vi "Sub-VI 1.vi"(0 "Select the chord name":string(combo), 1 "Display the musical notes":bool caption="Display the musical notes ?", 2 "Stop conversion":bool) -> (4 "B11":bool caption="Boolean", 8 "B1":bool caption="Boolean", 9 "N1":bool, 10 "B2":bool caption="Boolean", 11 "N2":bool, 12 "B3":bool caption="Boolean", 13 "N3":bool, 14 "B4":bool caption="Boolean", 15 "N4":bool, 16 "B5":bool caption="Boolean", 17 "N5":bool, 18 "B6":bool caption="Boolean", 19 "N6":bool, 20 "B7":bool caption="Boolean", 21 "B8":bool caption="Boolean", 22 "B9":bool caption="Boolean", 23 "B10":bool caption="Boolean", 26 "N7":bool, 27 "N8":bool)   [LabVIEW 2019]
panel:
  # "CHORDS BOX"
  # "Welcome \ndear apprentices"
  # "This App, tailor-made for you, has magic power. Which ?  \n\nThat of making you travel in the shoes \nof one of the greatest pianists of all time :"
  # "NOTES PLAYED BOX"
  # "3"
  # "4"
  # "5"
  # "6"
  # "7"
  # "1"
  # "2"
  # "8"
  # "Sir Elton John."
  # "Let yourself \nbe transported by its chords !"
  # "2"
  # "3"
  # "4"
  # "5"
  # "6"
  # "8"
  # "1"
  # "7"
  # "9"
  # "10"
  # "11"
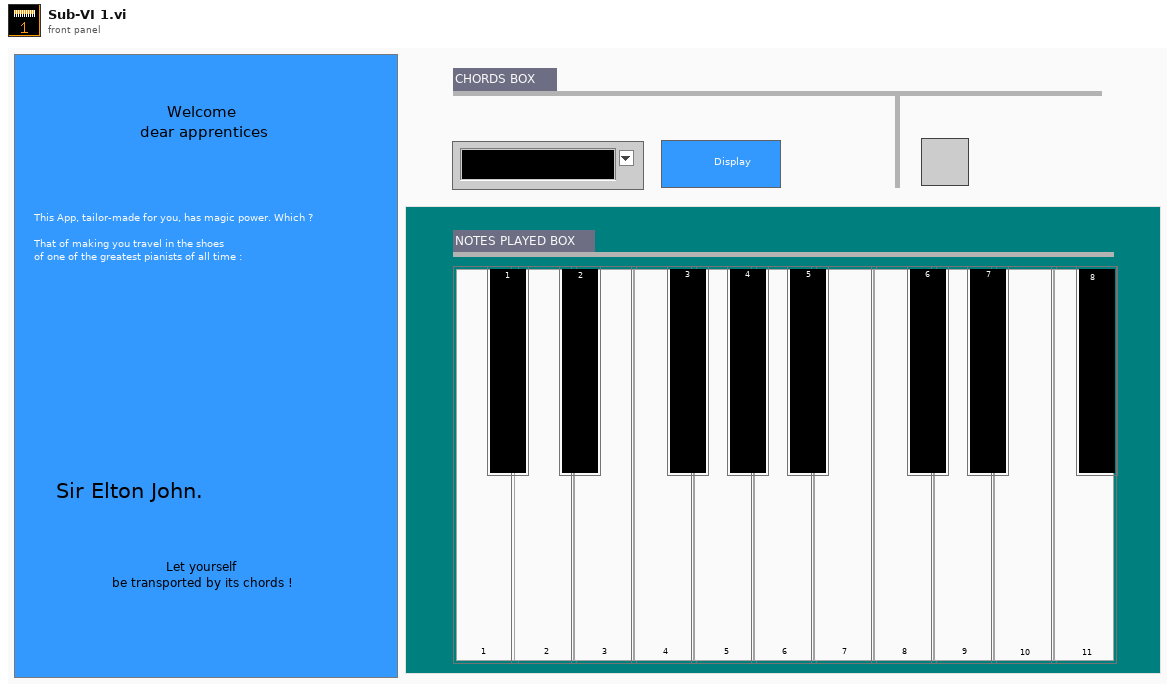
[diagram p1: front panel]
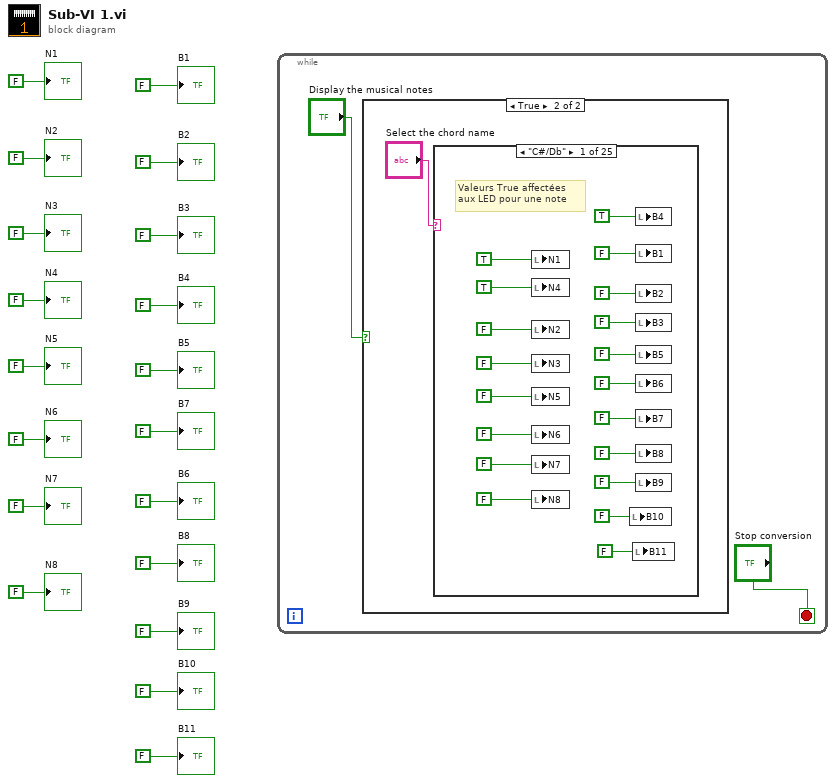
[diagram p0: block diagram]
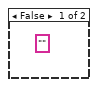
[diagram p2: hidden frame]
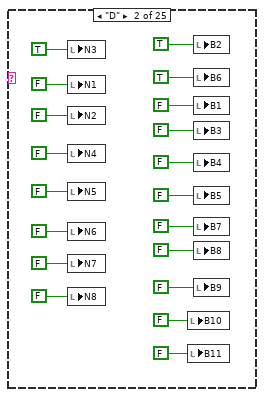
[diagram p3: hidden frame]
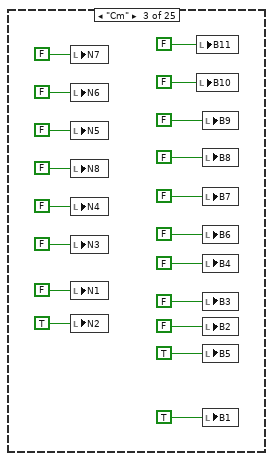
[diagram p4: hidden frame]
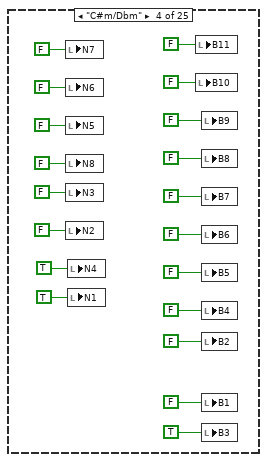
[diagram p5: hidden frame]
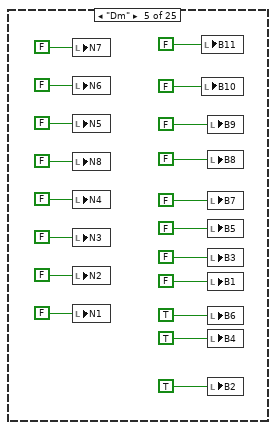
[diagram p6: hidden frame]
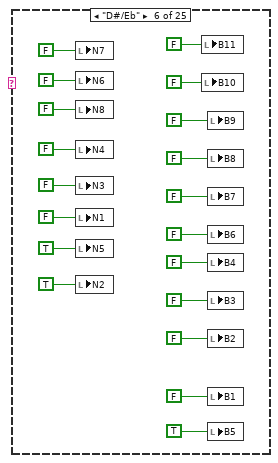
[diagram p7: hidden frame]
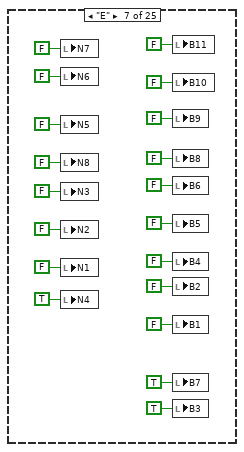
[diagram p8: hidden frame]
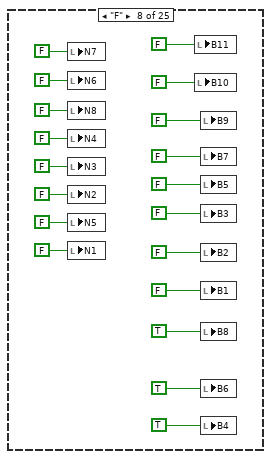
[diagram p9: hidden frame]
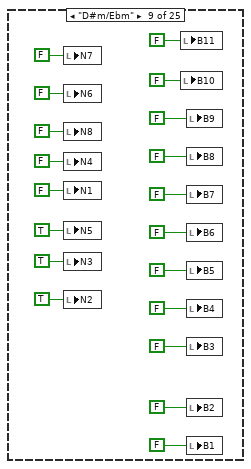
[diagram p10: hidden frame]
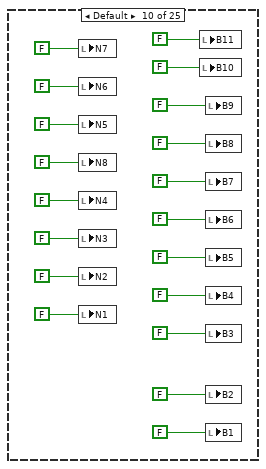
[diagram p11: hidden frame]
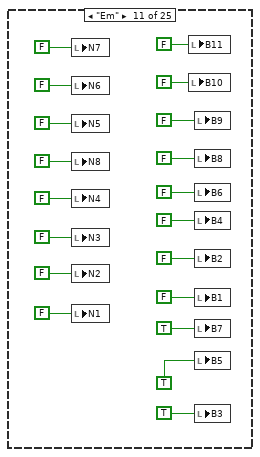
[diagram p12: hidden frame]
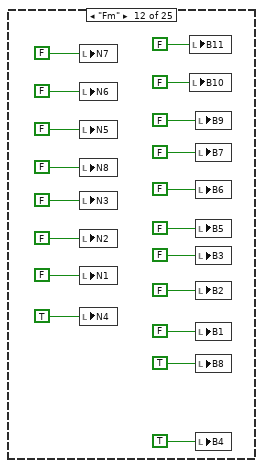
[diagram p13: hidden frame]
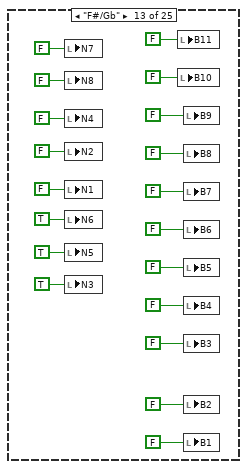
[diagram p14: hidden frame]
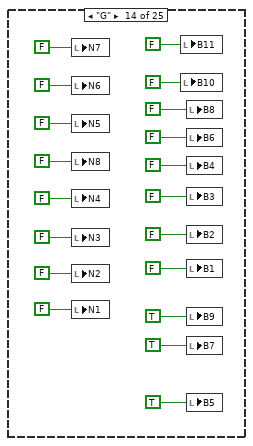
[diagram p15: hidden frame]
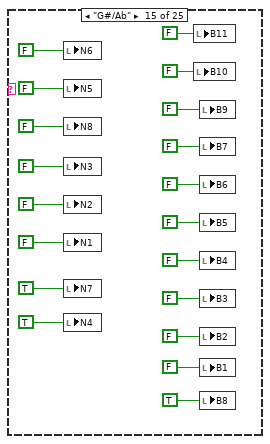
[diagram p16: hidden frame]
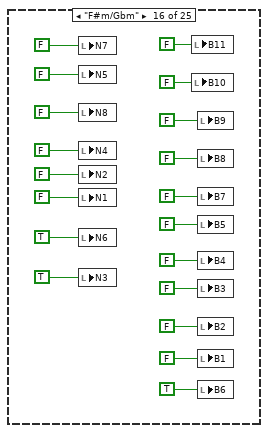
[diagram p17: hidden frame]
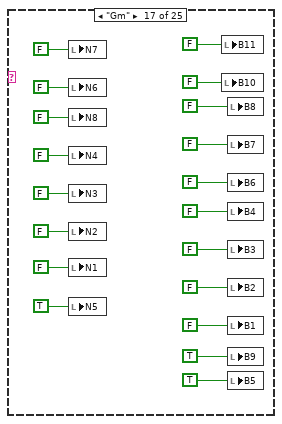
[diagram p18: hidden frame]
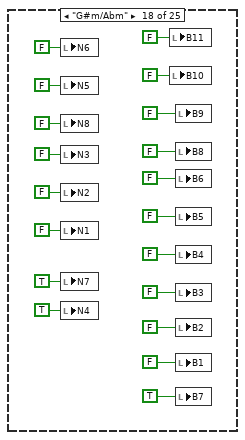
[diagram p19: hidden frame]
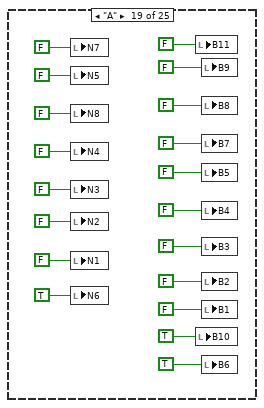
[diagram p20: hidden frame]
diagram:
  n1 = while {
    stop <- "Stop conversion" stop-if-true
    n2 = case shown="True" "Display the musical notes" {
      frame False {
        (unwired) ""
      }
      frame True {
        n3 = case shown="\"C#/Db\"" "Select the chord name" {
          frame "C#/Db" {
            # "Valeurs True affectées\naux LED pour une note"
            n4 = local write "N1"(TRUE) -> ()
            n5 = local write "N4"(TRUE) -> ()
            n6 = local write "N2"(FALSE) -> ()
            n7 = local write "N3"(FALSE) -> ()
            n8 = local write "N5"(FALSE) -> ()
            n9 = local write "N6"(FALSE) -> ()
            n10 = local write "N7"(FALSE) -> ()
            n11 = local write "N8"(FALSE) -> ()
            n12 = local write "B10"(FALSE) -> ()
            n13 = local write "B11"(FALSE) -> ()
            n14 = local write "B4"(TRUE) -> ()
            n15 = local write "B1"(FALSE) -> ()
            n16 = local write "B2"(FALSE) -> ()
            n17 = local write "B3"(FALSE) -> ()
            n18 = local write "B5"(FALSE) -> ()
            n19 = local write "B6"(FALSE) -> ()
            n20 = local write "B7"(FALSE) -> ()
            n21 = local write "B8"(FALSE) -> ()
            n22 = local write "B9"(FALSE) -> ()
          }
          frame "D" {
            n23 = local write "N3"(TRUE) -> ()
            n24 = local write "N1"(FALSE) -> ()
            n25 = local write "N2"(FALSE) -> ()
            n26 = local write "N4"(FALSE) -> ()
            n27 = local write "N5"(FALSE) -> ()
            n28 = local write "N6"(FALSE) -> ()
            n29 = local write "N7"(FALSE) -> ()
            n30 = local write "N8"(FALSE) -> ()
            n31 = local write "B10"(FALSE) -> ()
            n32 = local write "B11"(FALSE) -> ()
            n33 = local write "B2"(TRUE) -> ()
            n34 = local write "B6"(TRUE) -> ()
            n35 = local write "B1"(FALSE) -> ()
            n36 = local write "B3"(FALSE) -> ()
            n37 = local write "B4"(FALSE) -> ()
            n38 = local write "B5"(FALSE) -> ()
            n39 = local write "B7"(FALSE) -> ()
            n40 = local write "B8"(FALSE) -> ()
            n41 = local write "B9"(FALSE) -> ()
          }
          frame "Cm" {
            n42 = local write "N7"(FALSE) -> ()
            n43 = local write "N6"(FALSE) -> ()
            n44 = local write "N5"(FALSE) -> ()
            n45 = local write "N8"(FALSE) -> ()
            n46 = local write "N4"(FALSE) -> ()
            n47 = local write "N3"(FALSE) -> ()
            n48 = local write "N1"(FALSE) -> ()
            n49 = local write "N2"(TRUE) -> ()
            n50 = local write "B11"(FALSE) -> ()
            n51 = local write "B10"(FALSE) -> ()
            n52 = local write "B9"(FALSE) -> ()
            n53 = local write "B8"(FALSE) -> ()
            n54 = local write "B7"(FALSE) -> ()
            n55 = local write "B6"(FALSE) -> ()
            n56 = local write "B4"(FALSE) -> ()
            n57 = local write "B3"(FALSE) -> ()
            n58 = local write "B2"(FALSE) -> ()
            n59 = local write "B5"(TRUE) -> ()
            n60 = local write "B1"(TRUE) -> ()
          }
          frame "C#m/Dbm" {
            n61 = local write "N7"(FALSE) -> ()
            n62 = local write "N6"(FALSE) -> ()
            n63 = local write "N5"(FALSE) -> ()
            n64 = local write "N8"(FALSE) -> ()
            n65 = local write "N3"(FALSE) -> ()
            n66 = local write "N2"(FALSE) -> ()
            n67 = local write "N4"(TRUE) -> ()
            n68 = local write "N1"(TRUE) -> ()
            n69 = local write "B11"(FALSE) -> ()
            n70 = local write "B10"(FALSE) -> ()
            n71 = local write "B9"(FALSE) -> ()
            n72 = local write "B8"(FALSE) -> ()
            n73 = local write "B7"(FALSE) -> ()
            n74 = local write "B6"(FALSE) -> ()
            n75 = local write "B5"(FALSE) -> ()
            n76 = local write "B4"(FALSE) -> ()
            n77 = local write "B2"(FALSE) -> ()
            n78 = local write "B1"(FALSE) -> ()
            n79 = local write "B3"(TRUE) -> ()
          }
          frame "Dm" {
            n80 = local write "N7"(FALSE) -> ()
            n81 = local write "N6"(FALSE) -> ()
            n82 = local write "N5"(FALSE) -> ()
            n83 = local write "N8"(FALSE) -> ()
            n84 = local write "N4"(FALSE) -> ()
            n85 = local write "N3"(FALSE) -> ()
            n86 = local write "N2"(FALSE) -> ()
            n87 = local write "N1"(FALSE) -> ()
            n88 = local write "B11"(FALSE) -> ()
            n89 = local write "B10"(FALSE) -> ()
            n90 = local write "B9"(FALSE) -> ()
            n91 = local write "B8"(FALSE) -> ()
            n92 = local write "B7"(FALSE) -> ()
            n93 = local write "B5"(FALSE) -> ()
            n94 = local write "B3"(FALSE) -> ()
            n95 = local write "B1"(FALSE) -> ()
            n96 = local write "B6"(TRUE) -> ()
            n97 = local write "B4"(TRUE) -> ()
            n98 = local write "B2"(TRUE) -> ()
          }
          frame "D#/Eb" {
            n99 = local write "N7"(FALSE) -> ()
            n100 = local write "N6"(FALSE) -> ()
            n101 = local write "N8"(FALSE) -> ()
            n102 = local write "N4"(FALSE) -> ()
            n103 = local write "N3"(FALSE) -> ()
            n104 = local write "N1"(FALSE) -> ()
            n105 = local write "N5"(TRUE) -> ()
            n106 = local write "N2"(TRUE) -> ()
            n107 = local write "B11"(FALSE) -> ()
            n108 = local write "B10"(FALSE) -> ()
            n109 = local write "B9"(FALSE) -> ()
            n110 = local write "B8"(FALSE) -> ()
            n111 = local write "B7"(FALSE) -> ()
            n112 = local write "B6"(FALSE) -> ()
            n113 = local write "B4"(FALSE) -> ()
            n114 = local write "B3"(FALSE) -> ()
            n115 = local write "B2"(FALSE) -> ()
            n116 = local write "B1"(FALSE) -> ()
            n117 = local write "B5"(TRUE) -> ()
          }
          frame "E" {
            n118 = local write "N7"(FALSE) -> ()
            n119 = local write "N6"(FALSE) -> ()
            n120 = local write "N5"(FALSE) -> ()
            n121 = local write "N8"(FALSE) -> ()
            n122 = local write "N3"(FALSE) -> ()
            n123 = local write "N2"(FALSE) -> ()
            n124 = local write "N1"(FALSE) -> ()
            n125 = local write "N4"(TRUE) -> ()
            n126 = local write "B11"(FALSE) -> ()
            n127 = local write "B10"(FALSE) -> ()
            n128 = local write "B9"(FALSE) -> ()
            n129 = local write "B8"(FALSE) -> ()
            n130 = local write "B6"(FALSE) -> ()
            n131 = local write "B5"(FALSE) -> ()
            n132 = local write "B4"(FALSE) -> ()
            n133 = local write "B2"(FALSE) -> ()
            n134 = local write "B1"(FALSE) -> ()
            n135 = local write "B7"(TRUE) -> ()
            n136 = local write "B3"(TRUE) -> ()
          }
          frame "F" {
            n137 = local write "N7"(FALSE) -> ()
            n138 = local write "N6"(FALSE) -> ()
            n139 = local write "N8"(FALSE) -> ()
            n140 = local write "N4"(FALSE) -> ()
            n141 = local write "N3"(FALSE) -> ()
            n142 = local write "N2"(FALSE) -> ()
            n143 = local write "N5"(FALSE) -> ()
            n144 = local write "N1"(FALSE) -> ()
            n145 = local write "B11"(FALSE) -> ()
            n146 = local write "B10"(FALSE) -> ()
            n147 = local write "B9"(FALSE) -> ()
            n148 = local write "B7"(FALSE) -> ()
            n149 = local write "B5"(FALSE) -> ()
            n150 = local write "B3"(FALSE) -> ()
            n151 = local write "B2"(FALSE) -> ()
            n152 = local write "B1"(FALSE) -> ()
            n153 = local write "B8"(TRUE) -> ()
            n154 = local write "B6"(TRUE) -> ()
            n155 = local write "B4"(TRUE) -> ()
          }
          frame "D#m/Ebm" {
            n156 = local write "N7"(FALSE) -> ()
            n157 = local write "N6"(FALSE) -> ()
            n158 = local write "N8"(FALSE) -> ()
            n159 = local write "N4"(FALSE) -> ()
            n160 = local write "N1"(FALSE) -> ()
            n161 = local write "N5"(TRUE) -> ()
            n162 = local write "N3"(TRUE) -> ()
            n163 = local write "N2"(TRUE) -> ()
            n164 = local write "B11"(FALSE) -> ()
            n165 = local write "B10"(FALSE) -> ()
            n166 = local write "B9"(FALSE) -> ()
            n167 = local write "B8"(FALSE) -> ()
            n168 = local write "B7"(FALSE) -> ()
            n169 = local write "B6"(FALSE) -> ()
            n170 = local write "B5"(FALSE) -> ()
            n171 = local write "B4"(FALSE) -> ()
            n172 = local write "B3"(FALSE) -> ()
            n173 = local write "B2"(FALSE) -> ()
            n174 = local write "B1"(FALSE) -> ()
          }
          frame Default {
            n175 = local write "N7"(FALSE) -> ()
            n176 = local write "N6"(FALSE) -> ()
            n177 = local write "N5"(FALSE) -> ()
            n178 = local write "N8"(FALSE) -> ()
            n179 = local write "N4"(FALSE) -> ()
            n180 = local write "N3"(FALSE) -> ()
            n181 = local write "N2"(FALSE) -> ()
            n182 = local write "N1"(FALSE) -> ()
            n183 = local write "B11"(FALSE) -> ()
            n184 = local write "B10"(FALSE) -> ()
            n185 = local write "B9"(FALSE) -> ()
            n186 = local write "B8"(FALSE) -> ()
            n187 = local write "B7"(FALSE) -> ()
            n188 = local write "B6"(FALSE) -> ()
            n189 = local write "B5"(FALSE) -> ()
            n190 = local write "B4"(FALSE) -> ()
            n191 = local write "B3"(FALSE) -> ()
            n192 = local write "B2"(FALSE) -> ()
            n193 = local write "B1"(FALSE) -> ()
          }
          frame "Em" {
            n194 = local write "N7"(FALSE) -> ()
            n195 = local write "N6"(FALSE) -> ()
            n196 = local write "N5"(FALSE) -> ()
            n197 = local write "N8"(FALSE) -> ()
            n198 = local write "N4"(FALSE) -> ()
            n199 = local write "N3"(FALSE) -> ()
            n200 = local write "N2"(FALSE) -> ()
            n201 = local write "N1"(FALSE) -> ()
            n202 = local write "B11"(FALSE) -> ()
            n203 = local write "B10"(FALSE) -> ()
            n204 = local write "B9"(FALSE) -> ()
            n205 = local write "B8"(FALSE) -> ()
            n206 = local write "B6"(FALSE) -> ()
            n207 = local write "B4"(FALSE) -> ()
            n208 = local write "B2"(FALSE) -> ()
            n209 = local write "B1"(FALSE) -> ()
            n210 = local write "B7"(TRUE) -> ()
            n211 = local write "B5"(TRUE) -> ()
            n212 = local write "B3"(TRUE) -> ()
          }
          frame "Fm" {
            n213 = local write "N7"(FALSE) -> ()
            n214 = local write "N6"(FALSE) -> ()
            n215 = local write "N5"(FALSE) -> ()
            n216 = local write "N8"(FALSE) -> ()
            n217 = local write "N3"(FALSE) -> ()
            n218 = local write "N2"(FALSE) -> ()
            n219 = local write "N1"(FALSE) -> ()
            n220 = local write "N4"(TRUE) -> ()
            n221 = local write "B11"(FALSE) -> ()
            n222 = local write "B10"(FALSE) -> ()
            n223 = local write "B9"(FALSE) -> ()
            n224 = local write "B7"(FALSE) -> ()
            n225 = local write "B6"(FALSE) -> ()
            n226 = local write "B5"(FALSE) -> ()
            n227 = local write "B3"(FALSE) -> ()
            n228 = local write "B2"(FALSE) -> ()
            n229 = local write "B1"(FALSE) -> ()
            n230 = local write "B8"(TRUE) -> ()
            n231 = local write "B4"(TRUE) -> ()
          }
          frame "F#/Gb" {
            n232 = local write "N7"(FALSE) -> ()
            n233 = local write "N8"(FALSE) -> ()
            n234 = local write "N4"(FALSE) -> ()
            n235 = local write "N2"(FALSE) -> ()
            n236 = local write "N1"(FALSE) -> ()
            n237 = local write "N6"(TRUE) -> ()
            n238 = local write "N5"(TRUE) -> ()
            n239 = local write "N3"(TRUE) -> ()
            n240 = local write "B11"(FALSE) -> ()
            n241 = local write "B10"(FALSE) -> ()
            n242 = local write "B9"(FALSE) -> ()
            n243 = local write "B8"(FALSE) -> ()
            n244 = local write "B7"(FALSE) -> ()
            n245 = local write "B6"(FALSE) -> ()
            n246 = local write "B5"(FALSE) -> ()
            n247 = local write "B4"(FALSE) -> ()
            n248 = local write "B3"(FALSE) -> ()
            n249 = local write "B2"(FALSE) -> ()
            n250 = local write "B1"(FALSE) -> ()
          }
          frame "G" {
            n251 = local write "N7"(FALSE) -> ()
            n252 = local write "N6"(FALSE) -> ()
            n253 = local write "N5"(FALSE) -> ()
            n254 = local write "N8"(FALSE) -> ()
            n255 = local write "N4"(FALSE) -> ()
            n256 = local write "N3"(FALSE) -> ()
            n257 = local write "N2"(FALSE) -> ()
            n258 = local write "N1"(FALSE) -> ()
            n259 = local write "B11"(FALSE) -> ()
            n260 = local write "B10"(FALSE) -> ()
            n261 = local write "B8"(FALSE) -> ()
            n262 = local write "B6"(FALSE) -> ()
            n263 = local write "B4"(FALSE) -> ()
            n264 = local write "B3"(FALSE) -> ()
            n265 = local write "B2"(FALSE) -> ()
            n266 = local write "B1"(FALSE) -> ()
            n267 = local write "B9"(TRUE) -> ()
            n268 = local write "B7"(TRUE) -> ()
            n269 = local write "B5"(TRUE) -> ()
          }
          frame "G#/Ab" {
            n270 = local write "N6"(FALSE) -> ()
            n271 = local write "N5"(FALSE) -> ()
            n272 = local write "N8"(FALSE) -> ()
            n273 = local write "N3"(FALSE) -> ()
            n274 = local write "N2"(FALSE) -> ()
            n275 = local write "N1"(FALSE) -> ()
            n276 = local write "N7"(TRUE) -> ()
            n277 = local write "N4"(TRUE) -> ()
            n278 = local write "B11"(FALSE) -> ()
            n279 = local write "B10"(FALSE) -> ()
            n280 = local write "B9"(FALSE) -> ()
            n281 = local write "B7"(FALSE) -> ()
            n282 = local write "B6"(FALSE) -> ()
            n283 = local write "B5"(FALSE) -> ()
            n284 = local write "B4"(FALSE) -> ()
            n285 = local write "B3"(FALSE) -> ()
            n286 = local write "B2"(FALSE) -> ()
            n287 = local write "B1"(FALSE) -> ()
            n288 = local write "B8"(TRUE) -> ()
          }
          frame "F#m/Gbm" {
            n289 = local write "N7"(FALSE) -> ()
            n290 = local write "N5"(FALSE) -> ()
            n291 = local write "N8"(FALSE) -> ()
            n292 = local write "N4"(FALSE) -> ()
            n293 = local write "N2"(FALSE) -> ()
            n294 = local write "N1"(FALSE) -> ()
            n295 = local write "N6"(TRUE) -> ()
            n296 = local write "N3"(TRUE) -> ()
            n297 = local write "B11"(FALSE) -> ()
            n298 = local write "B10"(FALSE) -> ()
            n299 = local write "B9"(FALSE) -> ()
            n300 = local write "B8"(FALSE) -> ()
            n301 = local write "B7"(FALSE) -> ()
            n302 = local write "B5"(FALSE) -> ()
            n303 = local write "B4"(FALSE) -> ()
            n304 = local write "B3"(FALSE) -> ()
            n305 = local write "B2"(FALSE) -> ()
            n306 = local write "B1"(FALSE) -> ()
            n307 = local write "B6"(TRUE) -> ()
          }
          frame "Gm" {
            n308 = local write "N7"(FALSE) -> ()
            n309 = local write "N6"(FALSE) -> ()
            n310 = local write "N8"(FALSE) -> ()
            n311 = local write "N4"(FALSE) -> ()
            n312 = local write "N3"(FALSE) -> ()
            n313 = local write "N2"(FALSE) -> ()
            n314 = local write "N1"(FALSE) -> ()
            n315 = local write "N5"(TRUE) -> ()
            n316 = local write "B11"(FALSE) -> ()
            n317 = local write "B10"(FALSE) -> ()
            n318 = local write "B8"(FALSE) -> ()
            n319 = local write "B7"(FALSE) -> ()
            n320 = local write "B6"(FALSE) -> ()
            n321 = local write "B4"(FALSE) -> ()
            n322 = local write "B3"(FALSE) -> ()
            n323 = local write "B2"(FALSE) -> ()
            n324 = local write "B1"(FALSE) -> ()
            n325 = local write "B9"(TRUE) -> ()
            n326 = local write "B5"(TRUE) -> ()
          }
          frame "G#m/Abm" {
            n327 = local write "N6"(FALSE) -> ()
            n328 = local write "N5"(FALSE) -> ()
            n329 = local write "N8"(FALSE) -> ()
            n330 = local write "N3"(FALSE) -> ()
            n331 = local write "N2"(FALSE) -> ()
            n332 = local write "N1"(FALSE) -> ()
            n333 = local write "N7"(TRUE) -> ()
            n334 = local write "N4"(TRUE) -> ()
            n335 = local write "B11"(FALSE) -> ()
            n336 = local write "B10"(FALSE) -> ()
            n337 = local write "B9"(FALSE) -> ()
            n338 = local write "B8"(FALSE) -> ()
            n339 = local write "B6"(FALSE) -> ()
            n340 = local write "B5"(FALSE) -> ()
            n341 = local write "B4"(FALSE) -> ()
            n342 = local write "B3"(FALSE) -> ()
            n343 = local write "B2"(FALSE) -> ()
            n344 = local write "B1"(FALSE) -> ()
            n345 = local write "B7"(TRUE) -> ()
          }
          frame "A" {
            n346 = local write "N7"(FALSE) -> ()
            n347 = local write "N5"(FALSE) -> ()
            n348 = local write "N8"(FALSE) -> ()
            n349 = local write "N4"(FALSE) -> ()
            n350 = local write "N3"(FALSE) -> ()
            n351 = local write "N2"(FALSE) -> ()
            n352 = local write "N1"(FALSE) -> ()
            n353 = local write "N6"(TRUE) -> ()
            n354 = local write "B11"(FALSE) -> ()
            n355 = local write "B10"(TRUE) -> ()
            n356 = local write "B9"(FALSE) -> ()
            n357 = local write "B8"(FALSE) -> ()
            n358 = local write "B7"(FALSE) -> ()
            n359 = local write "B5"(FALSE) -> ()
            n360 = local write "B4"(FALSE) -> ()
            n361 = local write "B3"(FALSE) -> ()
            n362 = local write "B2"(FALSE) -> ()
            n363 = local write "B1"(FALSE) -> ()
            n364 = local write "B6"(TRUE) -> ()
          }
          frame "A#/Bb" {
            n365 = local write "N8"(FALSE) -> ()
            n366 = local write "N4"(FALSE) -> ()
            n367 = local write "N3"(FALSE) -> ()
            n368 = local write "N2"(FALSE) -> ()
            n369 = local write "N1"(FALSE) -> ()
            n370 = local write "N5"(TRUE) -> ()
            n371 = local write "B10"(FALSE) -> ()
            n372 = local write "B11"(TRUE) -> ()
            n373 = local write "B8"(FALSE) -> ()
            n374 = local write "B7"(FALSE) -> ()
            n375 = local write "B6"(FALSE) -> ()
            n376 = local write "B5"(FALSE) -> ()
            n377 = local write "B4"(FALSE) -> ()
            n378 = local write "B3"(FALSE) -> ()
            n379 = local write "B2"(FALSE) -> ()
            n380 = local write "B1"(FALSE) -> ()
            n381 = local write "B9"(TRUE) -> ()
          }
          frame "B" {
            n382 = local write "N6"(FALSE) -> ()
            n383 = local write "N5"(FALSE) -> ()
            n384 = local write "N4"(FALSE) -> ()
            n385 = local write "N3"(FALSE) -> ()
            n386 = local write "N2"(FALSE) -> ()
            n387 = local write "N1"(FALSE) -> ()
            n388 = local write "N7"(TRUE) -> ()
            n389 = local write "N8"(TRUE) -> ()
            n390 = local write "B11"(FALSE) -> ()
            n391 = local write "B10"(FALSE) -> ()
            n392 = local write "B9"(FALSE) -> ()
            n393 = local write "B8"(FALSE) -> ()
            n394 = local write "B6"(FALSE) -> ()
            n395 = local write "B5"(FALSE) -> ()
            n396 = local write "B4"(FALSE) -> ()
            n397 = local write "B3"(FALSE) -> ()
            n398 = local write "B2"(FALSE) -> ()
            n399 = local write "B1"(FALSE) -> ()
            n400 = local write "B7"(TRUE) -> ()
          }
          frame "Am" {
            n401 = local write "N7"(FALSE) -> ()
            n402 = local write "N6"(FALSE) -> ()
            n403 = local write "N5"(FALSE) -> ()
            n404 = local write "N8"(FALSE) -> ()
            n405 = local write "N4"(FALSE) -> ()
            n406 = local write "N3"(FALSE) -> ()
            n407 = local write "N2"(FALSE) -> ()
            n408 = local write "N1"(FALSE) -> ()
            n409 = local write "B11"(FALSE) -> ()
            n410 = local write "B10"(TRUE) -> ()
            n411 = local write "B9"(FALSE) -> ()
            n412 = local write "B7"(FALSE) -> ()
            n413 = local write "B5"(FALSE) -> ()
            n414 = local write "B4"(FALSE) -> ()
            n415 = local write "B3"(FALSE) -> ()
            n416 = local write "B2"(FALSE) -> ()
            n417 = local write "B1"(FALSE) -> ()
            n418 = local write "B8"(TRUE) -> ()
            n419 = local write "B6"(TRUE) -> ()
          }
          frame "A#m/Bbm" {
            n420 = local write "N7"(FALSE) -> ()
            n421 = local write "N8"(FALSE) -> ()
            n422 = local write "N4"(FALSE) -> ()
            n423 = local write "N3"(FALSE) -> ()
            n424 = local write "N2"(FALSE) -> ()
            n425 = local write "N1"(FALSE) -> ()
            n426 = local write "N6"(TRUE) -> ()
            n427 = local write "N5"(TRUE) -> ()
            n428 = local write "B10"(FALSE) -> ()
            n429 = local write "B11"(TRUE) -> ()
            n430 = local write "B9"(FALSE) -> ()
            n431 = local write "B8"(FALSE) -> ()
            n432 = local write "B7"(FALSE) -> ()
            n433 = local write "B6"(FALSE) -> ()
            n434 = local write "B5"(FALSE) -> ()
            n435 = local write "B4"(FALSE) -> ()
            n436 = local write "B3"(FALSE) -> ()
            n437 = local write "B2"(FALSE) -> ()
            n438 = local write "B1"(FALSE) -> ()
          }
          frame "Bm" {
            n439 = local write "N7"(FALSE) -> ()
            n440 = local write "N6"(FALSE) -> ()
            n441 = local write "N5"(FALSE) -> ()
            n442 = local write "N4"(FALSE) -> ()
            n443 = local write "N3"(FALSE) -> ()
            n444 = local write "N2"(FALSE) -> ()
            n445 = local write "N1"(FALSE) -> ()
            n446 = local write "N8"(TRUE) -> ()
            n447 = local write "B11"(FALSE) -> ()
            n448 = local write "B10"(FALSE) -> ()
            n449 = local write "B8"(FALSE) -> ()
            n450 = local write "B6"(FALSE) -> ()
            n451 = local write "B5"(FALSE) -> ()
            n452 = local write "B4"(FALSE) -> ()
            n453 = local write "B3"(FALSE) -> ()
            n454 = local write "B2"(FALSE) -> ()
            n455 = local write "B1"(FALSE) -> ()
            n456 = local write "B9"(TRUE) -> ()
            n457 = local write "B7"(TRUE) -> ()
          }
          frame "C" {
            n458 = local write "N7"(FALSE) -> ()
            n459 = local write "N6"(FALSE) -> ()
            n460 = local write "N5"(FALSE) -> ()
            n461 = local write "N8"(FALSE) -> ()
            n462 = local write "N4"(FALSE) -> ()
            n463 = local write "N3"(FALSE) -> ()
            n464 = local write "N2"(FALSE) -> ()
            n465 = local write "N1"(FALSE) -> ()
            n466 = local write "B11"(FALSE) -> ()
            n467 = local write "B10"(FALSE) -> ()
            n468 = local write "B9"(FALSE) -> ()
            n469 = local write "B8"(FALSE) -> ()
            n470 = local write "B7"(FALSE) -> ()
            n471 = local write "B6"(FALSE) -> ()
            n472 = local write "B4"(FALSE) -> ()
            n473 = local write "B2"(FALSE) -> ()
            n474 = local write "B5"(TRUE) -> ()
            n475 = local write "B3"(TRUE) -> ()
            n476 = local write "B1"(TRUE) -> ()
          }
        }
      }
    }
  }
  "B1" <- FALSE
  "N1" <- FALSE
  "B2" <- FALSE
  "B3" <- FALSE
  "B4" <- FALSE
  "B5" <- FALSE
  "B6" <- FALSE
  "B7" <- FALSE
  "B8" <- FALSE
  "B9" <- FALSE
  "B10" <- FALSE
  "B11" <- FALSE
  "N2" <- FALSE
  "N3" <- FALSE
  "N4" <- FALSE
  "N8" <- FALSE
  "N5" <- FALSE
  "N6" <- FALSE
  "N7" <- FALSE
